vi "Create Circular Marker.vi"(5 "Y Radius":dbl=100.0 format="%#_13g", 7 "X Radius":dbl=100.0 format="%#_13g", 8 "Y Center":dbl=100.0 format="%#_13g", 9 "X Center":dbl=100.0 format="%#_13g", 11 "Number of Points":i32=505) -> (3 "XY Graph":cluster{dbl[], dbl[]}(graph))   [LabVIEW 2013]
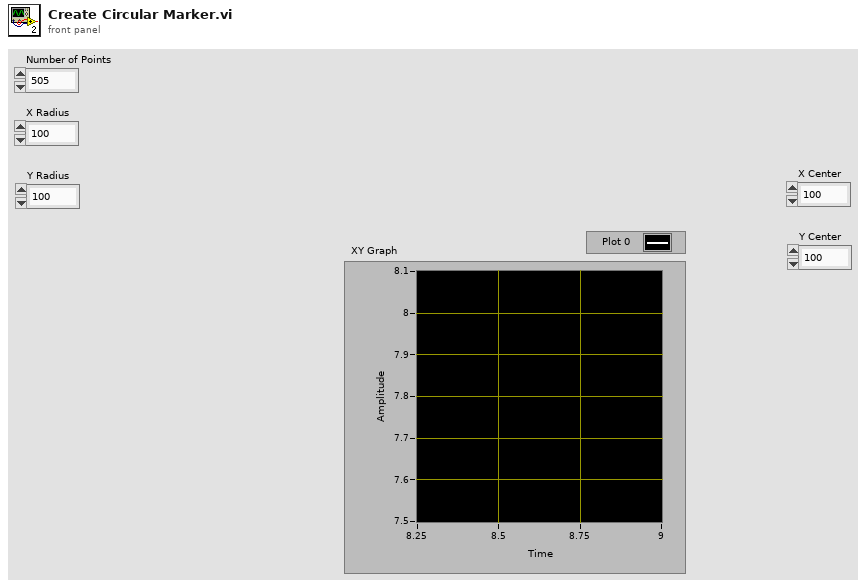
[diagram p1: front panel]
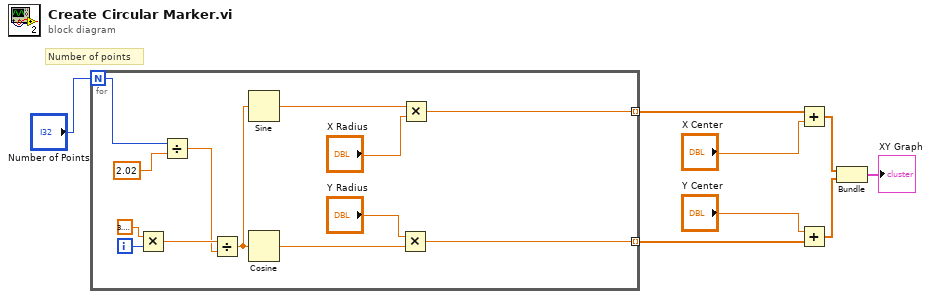
[diagram p0: block diagram]
diagram:
  # "Number of points"
  n1 = for {
    N: "Number of Points" -> [w13]
    tunnel: [w14] -> w6 mode=indexing
    tunnel: [w15] -> w5 mode=indexing
    i -> [w20]
    n2 = Multiply(x=3.141592653589793, y=w20) -> (x*y=w19:dbl)
    n3 = Divide(x=w13, y=2.02) -> (x/y=w12:dbl)
    n4 = Divide(x=w19, y=w12) -> (x/y=w18:dbl)
    n5 = Sine(x=w18) -> (sin(x)=w17:dbl)
    n6 = Cosine(x=w18) -> (cos(x)=w16:dbl)
    n7 = Multiply(x="Y Radius", y=w16) -> (x*y=w15:dbl)
    n8 = Multiply(x=w17, y="X Radius") -> (x*y=w14:dbl)
  }
  n9 = Add(x=w6, y="X Center") -> (x+y=w4:dbl[])
  n10 = Add(x="Y Center", y=w5) -> (x+y=w3:dbl[])
  n11 = Bundle(w4, w3) -> (→"XY Graph":cluster{dbl[], dbl[]})  [unwired: 1 in]
